vi "onboard.LED.vi"(11 "OnBoard.LED[3:0]":fxp<+,4,4>) -> ()   [LabVIEW 2019]
uses:
  <vilib>/rvi/eio/common/nirviEmuTemplateMethod_errors.vi
  <vilib>/eio/EIONode/EIONode.xnode
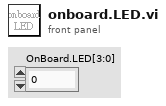
[diagram p1: front panel]
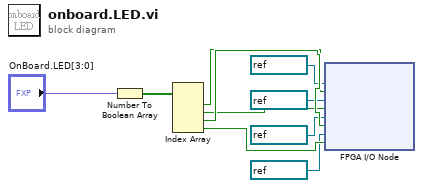
[diagram p0: block diagram]
diagram:
  n1 = Number To Boolean Array(number="OnBoard.LED[3:0]") -> (Boolean array=w9:bool[])
  n2 = Index Array(array=w9) -> (element #1=w5:bool, element #2=w6:bool, element #3=w7:bool, element #4=w8:bool)  [unwired: 4 in]
  n3 = xnode "FPGA I/O Node"("I/O Item"=w5, "FPGA I/O In"=refnum<k21> "LED0", "I/O Item"=w6, "FPGA I/O In"=refnum<k21> "LED1", "I/O Item"=w7, "FPGA I/O In"=refnum<k21> "LED2", "I/O Item"=w8, "FPGA I/O In"=refnum<k21> "LED3") -> ()  [unwired: 4 out]
